vi "DriveTeleopCommand.vi"(11 "Axes":dbl[](array[numeric])) -> ()   [LabVIEW 2017]
uses:
  DriveCommand.ctl
  RunMode.ctl
  Robot Global Data.vi
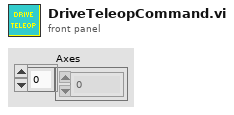
[diagram p1: front panel]
types:
  T1 = typedef "RunMode.ctl" = enum16{"Auto", "Teleop", "Disabled"}
  T2 = typedef "DriveCommand.ctl" = cluster{"LeftDriveMagnatude":dbl, "RightDriveMagnatude":dbl, "Mode":T1}
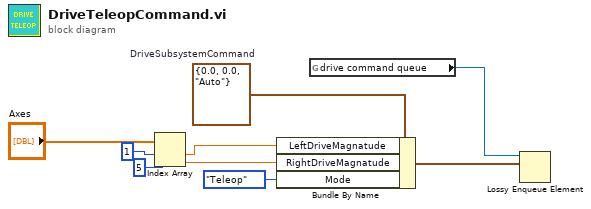
[diagram p0: block diagram]
diagram:
  w6 = T2 {"LeftDriveMagnatude"=0.0, "RightDriveMagnatude"=0.0, "Mode"=enum."Auto"}  # DriveSubsystemCommand
  n1 = Index Array(array="Axes", index #1=1 ("index"), index #2=5 ("index")) -> (element #1=w8:dbl, element #2=w9:dbl)
  n2 = Bundle By Name(cluster=w6, "LeftDriveMagnatude"=w8, "RightDriveMagnatude"=w9, "Mode"=RunMode."Teleop") -> (w7:T2)
  n3 = global read "Robot Global Data.vi" "drive command queue"() -> (w1:refnum<queue>)
  n4 = Lossy Enqueue Element(queue=w1, element=w7) -> ()  [unwired: 1 in, 4 out]
